vi "Configure Math Function (Bus).vi"(4 "Math Function Index (1: Math Function 1)":i32(ring)=1 items=["Math Function 1"=1, "Math Function 2"=2, "Math Function 3"=3, "Math Function 4"=4], 5 "Vertical Units (0: Volt)":i32(ring) items=["Volt", "Ampere", "None"], 6 "Origin Bus Data (0)":dbl, 7 "Bus Data Increment (0.001)":dbl=0.001, 8 "error in (no error)":errorcluster, 9 "Clock Signal Slope (1: Positive)":i32(ring)=1 items=["Negative", "Positive", "Either"], 10 "Clock Signal Source (0)":i32, 11 "VISA resource name":refnum<visa-resource-name>) -> (0 "error out":errorcluster, 3 "VISA resource name out":refnum<visa-resource-name>)   [LabVIEW 2015, in "Agilent 2000 3000 X-Series.lvlib"]
doc: "Configures the BUS math function.\n\n<B>Note(s):</B>\nThis function is available only with the DSOX3ADVMATH advanced math license."
uses:
  <instrlib>/Agilent 2000 3000 X-Series/Agilent 2000 3000 X-Series.lvlib
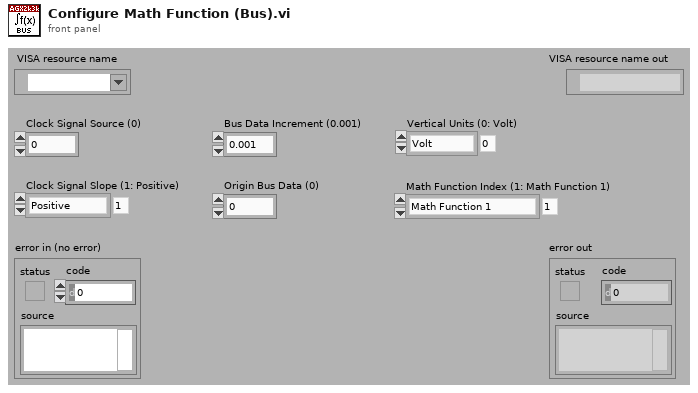
[diagram p1: front panel]
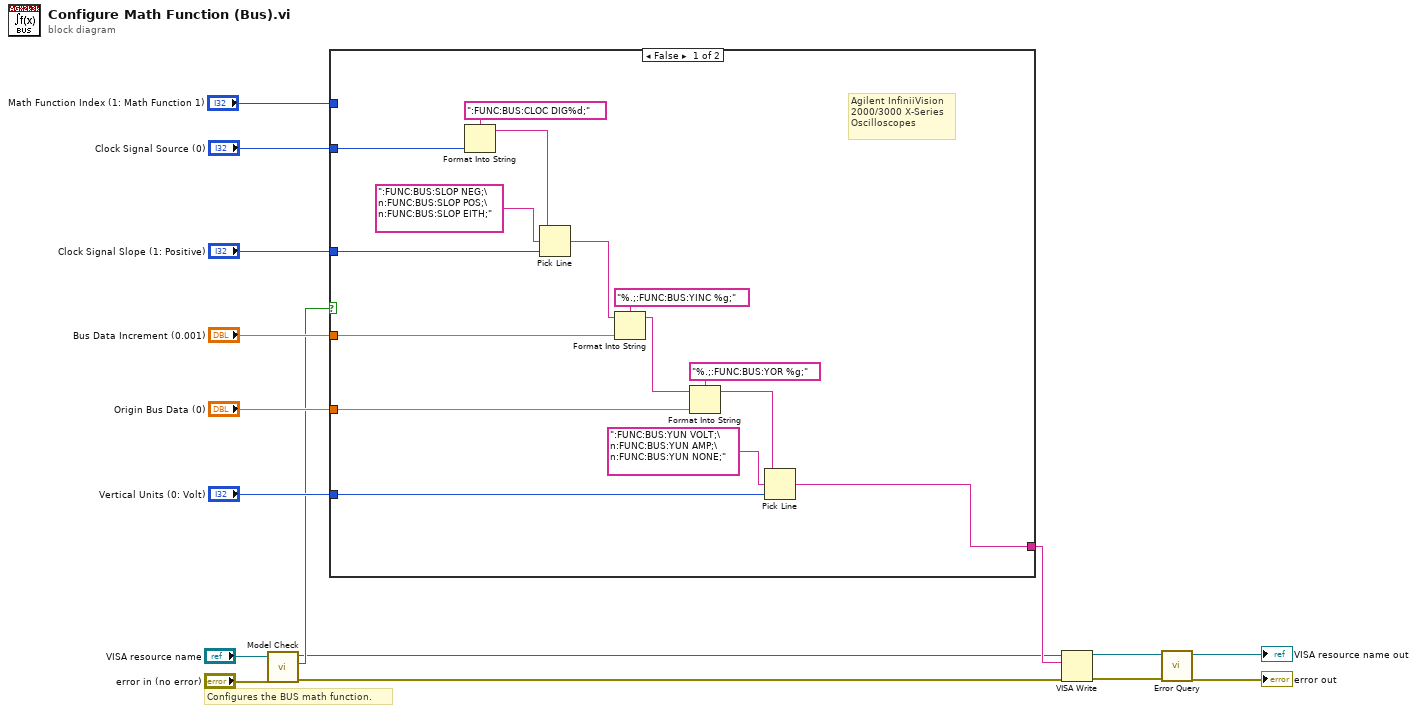
[diagram p0: block diagram]
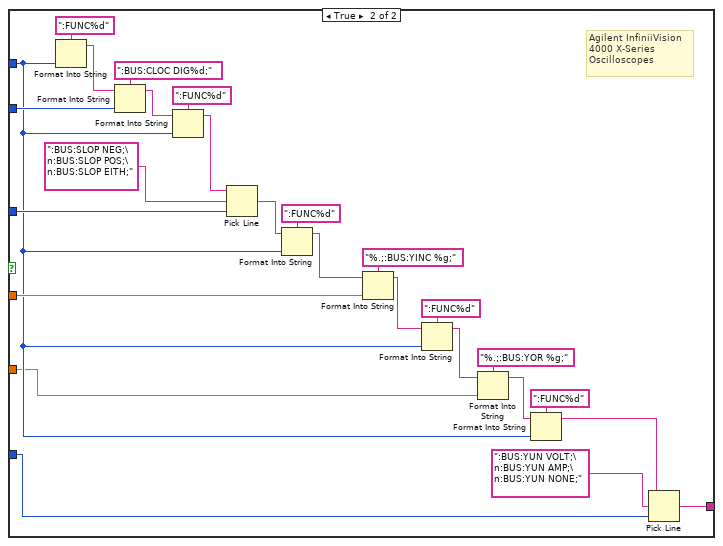
[diagram p2: hidden frame]
diagram:
  # "Configures the BUS math function."
  n1 = call <instrlib>:"Model Check.vi"("error in (no error)"="error in (no error)", "VISA resource name"="VISA resource name") -> ("error out"=w1:errorcluster, "Not 2000 or 3000 Series"=w5:bool, "VISA resource name out"=w2:refnum<visa-resource-name>)  [unwired: 7 out]
  n2 = case shown="False" w5 {
    tunnel: "Clock Signal Source (0)" -> [w22 w50]
    tunnel: "Clock Signal Slope (1: Positive)" -> [w21 w47]
    tunnel: "Bus Data Increment (0.001)" -> [w20 w42]
    tunnel: "Origin Bus Data (0)" -> [w19 w32]
    tunnel: "Vertical Units (0: Volt)" -> [w18 w41]
    tunnel: "Math Function Index (1: Math Function 1)" -> [_ w33]
    tunnel: [w17 w34] -> w6
    frame False {
      # "Agilent InfiniiVision\n2000/3000 X-Series\nOscilloscopes"
      n3 = Format Into String(format string=":FUNC:BUS:CLOC DIG%d;", w22) -> (resulting string=w25:string)  [unwired: 2 in, 1 out]
      n4 = Pick Line(string ("")=w25, multi-line string=":FUNC:BUS:SLOP NEG;\n:FUNC:BUS:SLOP POS;\n:FUNC:BUS:SLOP EITH;", line index=w21) -> (output string=w26:string)
      n5 = Format Into String(format string="%.;:FUNC:BUS:YINC %g;", initial string=w26, w20) -> (resulting string=w28:string)  [unwired: 1 in, 1 out]
      n6 = Format Into String(format string="%.;:FUNC:BUS:YOR %g;", initial string=w28, w19) -> (resulting string=w31:string)  [unwired: 1 in, 1 out]
      n7 = Pick Line(string ("")=w31, multi-line string=":FUNC:BUS:YUN VOLT;\n:FUNC:BUS:YUN AMP;\n:FUNC:BUS:YUN NONE;", line index=w18) -> (output string=w17:string)
    }
    frame True {
      # "Agilent InfiniiVision\n4000 X-Series\nOscilloscopes"
      n8 = Format Into String(format string=":FUNC%d", w33) -> (resulting string=w51:string)  [unwired: 2 in, 1 out]
      n9 = Format Into String(format string=":BUS:CLOC DIG%d;", initial string=w51, w50) -> (resulting string=w48:string)  [unwired: 1 in, 1 out]
      n10 = Format Into String(format string=":FUNC%d", initial string=w48, w33) -> (resulting string=w46:string)  [unwired: 1 in, 1 out]
      n11 = Pick Line(string ("")=w46, multi-line string=":BUS:SLOP NEG;\n:BUS:SLOP POS;\n:BUS:SLOP EITH;", line index=w47) -> (output string=w44:string)
      n12 = Format Into String(format string=":FUNC%d", initial string=w44, w33) -> (resulting string=w43:string)  [unwired: 1 in, 1 out]
      n13 = Format Into String(format string="%.;:BUS:YINC %g;", initial string=w43, w42) -> (resulting string=w39:string)  [unwired: 1 in, 1 out]
      n14 = Format Into String(format string=":FUNC%d", initial string=w39, w33) -> (resulting string=w38:string)  [unwired: 1 in, 1 out]
      n15 = Format Into String(format string="%.;:BUS:YOR %g;", initial string=w38, w32) -> (resulting string=w36:string)  [unwired: 1 in, 1 out]
      n16 = Format Into String(format string=":FUNC%d", initial string=w36, w33) -> (resulting string=w35:string)  [unwired: 1 in, 1 out]
      n17 = Pick Line(string ("")=w35, multi-line string=":BUS:YUN VOLT;\n:BUS:YUN AMP;\n:BUS:YUN NONE;", line index=w41) -> (output string=w34:string)
    }
  }
  n18 = VISA Write(VISA resource name=w2, write buffer=w6, error in (no error)=w1) -> (VISA resource name out=w16:refnum<visa-resource-name>, error out=w15:errorcluster)  [unwired: 1 out]
  n19 = call <instrlib>:"Error Query.vi"("error in (no error)"=w15, "VISA resource name"=w16) -> ("error out"=→"error out":errorcluster, "VISA resource name out"=→"VISA resource name out":refnum<visa-resource-name>)  [unwired: 8 out]
